vi "Destroy Loader.vi"(6 "timeout (ms)":i32=5000, 8 "error in":errorcluster, 11 "gRPC ID in":T1) -> (0 "error out":errorcluster, 3 "gRPC ID out":T1)   [LabVIEW 2021, in "CIFPluginLoaderClientWrapper.lvlib"]
uses:
  CIFPluginLoaderClientWrapper.lvlib
  CIF_PluginLoader_client/CIF_PluginLoader_client.lvlib
  CIF_PluginLoader_client/RPC Messages/cif_pluginloader_DestroyRequest.ctl
  <vilib>/gRPC/LabVIEW gRPC Library/Shared/grpcId.ctl
  <vilib>/gRPC/LabVIEW gRPC Library/grpc-lvsupport-release.lvlib
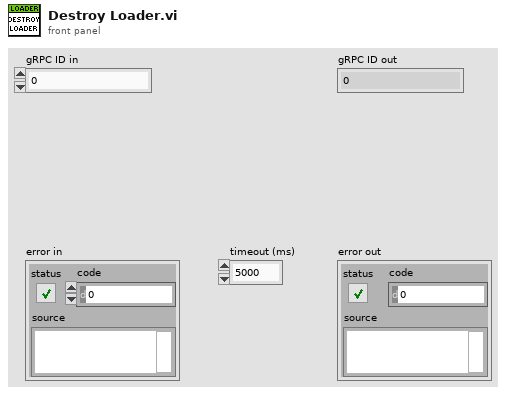
[diagram p1: front panel]
types:
  T1 = typedef "grpc-lvsupport-release.lvlib/grpcId.ctl" = u64
  T2 = typedef "CIF_PluginLoader_client.lvlib/cif_pluginloader_DestroyRequest.ctl" = cluster{"void":string}
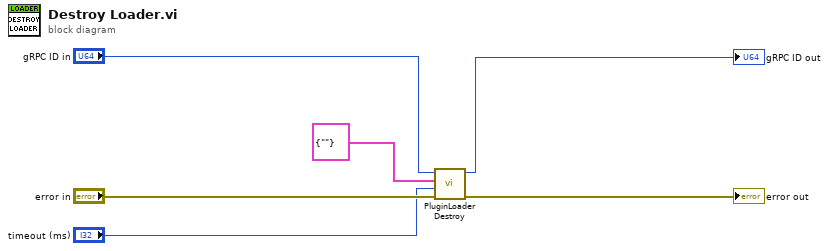
[diagram p0: block diagram]
diagram:
  n1 = call "PluginLoader Destroy.vi"("error in"="error in", "timeout (ms)"="timeout (ms)", "Request Data"=T2 {"void"=""}, "gRPC ID"="gRPC ID in") -> ("error out"=→"error out":errorcluster, "gRPC ID out"=→"gRPC ID out":T1)  [unwired: 5 in, 1 out]
